vi "GoTo PID vetor.vi"(8 "Position":dbl[](array[numeric]), 11 "Target":dbl[](array[numeric])) -> (3 "Velocity":dbl[](array[numeric]))   [LabVIEW 2016]
uses:
  <vilib>/Analysis/coordinate.llb/2D Cartesian Coordinate Rotation (Scalar).vi
  <vilib>/addons/control/pid/pid.llb/PID (DBL Array).vi
  <vilib>/Analysis/NI_AALPro.lvlib
  <vilib>/addons/control/pid/NI_PID_pid.lvlib
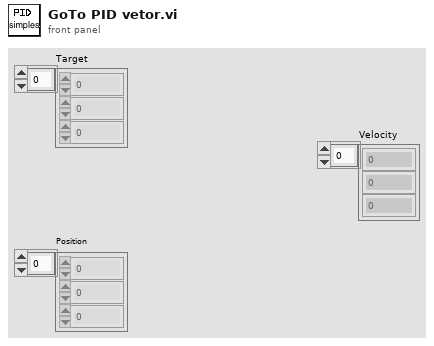
[diagram p1: front panel]
types:
  T1 = cluster{"proportional gain (Kc)":dbl, "integral time (Ti, min)":dbl, "derivative time (Td, min)":dbl}[]
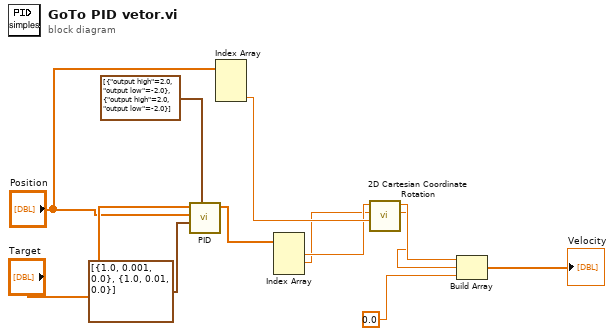
[diagram p0: block diagram]
diagram:
  n1 = call-poly <vilib>:"PID.vi"("output range"=cluster{"output high":dbl, "output low":dbl}[] [{"output high"=2.0, "output low"=-2.0}, {"output high"=2.0, "output low"=-2.0}], "PID gains"=T1 [{"proportional gain (Kc)"=1.0, "integral time (Ti, min)"=0.001, "derivative time (Td, min)"=0.0}, {"proportional gain (Kc)"=1.0, "integral time (Ti, min)"=0.01, "derivative time (Td, min)"=0.0}], "process variable"="Position", "setpoint"="Target") -> ("output"=w7:dbl[])  [unwired: 6 in, 1 out]
  n2 = Index Array(array="Position") -> (element #3=w8:dbl)  [unwired: 3 in, 2 out]
  n3 = Index Array(array=w7) -> (element #1=w3:dbl, element #2=w2:dbl)  [unwired: 3 in, 1 out]
  n4 = call-poly <vilib>:"2D Cartesian Coordinate Rotation.vi"("theta"=w8, "y"=w2, "x"=w3) -> ("y out"=w10:dbl, "x out"=w11:dbl)  [unwired: 6 in, 1 out]
  n5 = Build Array(w11, w10, 0.0 ("element")) -> (→"Velocity":dbl[])
